vi "Calibrate VNA.vi"(8 "error in (no error)":errorcluster, 9 "Cal kit type":enum16{"E-CAL", "Mechanical"}(ring), 10 "Calibration mode":enum16{"1 Port", "2  Port", "3 Port", "4 Port"}(ring), 11 "VNA-CMT S2 S4 in":refnum<class "VNA-CMT S2 S4.lvclass">) -> (0 "error out":errorcluster, 3 "VNA-CMT S2 S4 out":refnum<class "VNA-CMT S2 S4.lvclass">)   [LabVIEW 2020, in "VNA-CMT S2 S4.lvclass"]
uses:
  VNA-CMT S2 S4.lvclass
  Vector Network Analyzer.lvclass
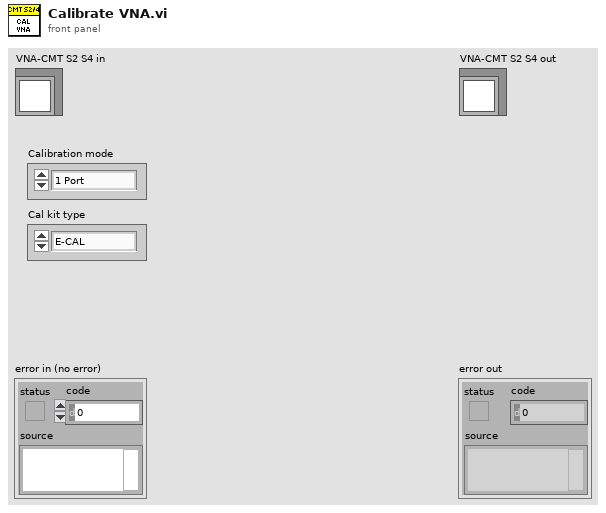
[diagram p1: front panel]
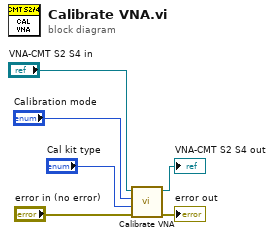
[diagram p0: block diagram]
diagram:
  n1 = call-parent "Calibrate VNA.vi"("error in (no error)"="error in (no error)", "Cal kit type"="Cal kit type", "Calibration mode"="Calibration mode", "Vector Network Analyzer in"="VNA-CMT S2 S4 in") -> ("error out"=→"error out":errorcluster, "Vector Network Analyzer out"=→"VNA-CMT S2 S4 out":refnum<class "VNA-CMT S2 S4.lvclass">)  [unwired: 6 in]
